vi "Array lezione operazioni.vi"() -> ()   [LabVIEW 2012]
panel:
  in  "Array":dbl[](array[numeric])
  in  "vet a":dbl[](array[numeric])=[1.0, 2.0, 3.0] format="%.2f"
  in  "vet b":dbl[](array[numeric]) format="%.2f"
  out "vet som":dbl[](array[numeric]) format="%.2f"
  in  "index select 2":i32=1
  out "index of elem.":i32=4
  in  "element":sgl format="%.2f"
  in  "start index":i32
  out "min index":i32=4
  out "min":sgl format="%.2f"
  out "max index":i32=4
  out "max":sgl format="%.2f"
  out "array cast":sgl[](array[numeric]) format="%.2f"
  in  "new element2":sgl=-2.0 format="%.2f"
  in  "new element1":sgl=3.0 format="%.2f"
  in  "lenght":i32=2
  out "array subset":sgl[](array[numeric]) format="%.2f"
  out "array out":sgl[](array[numeric]) format="%.2f"
  in  "element repl":sgl format="%.2f"
  in  "index select":i32=2
  out "element":sgl format="%.2f"
  in  "index":i32=3
  out "dim":i32=4
  in  "array in":sgl[](array[numeric])=[2.0, 4.0, 6.0, 8.0] format="%.2f"
  # "Funzioni che operano sugli array"
  # "Array Size"
  # "Index Array"
  # "Replace Array Element"
  # "Array Subset"
  # "Build Array"
  # "Array Max & Min"
  # "Search 1D Array"
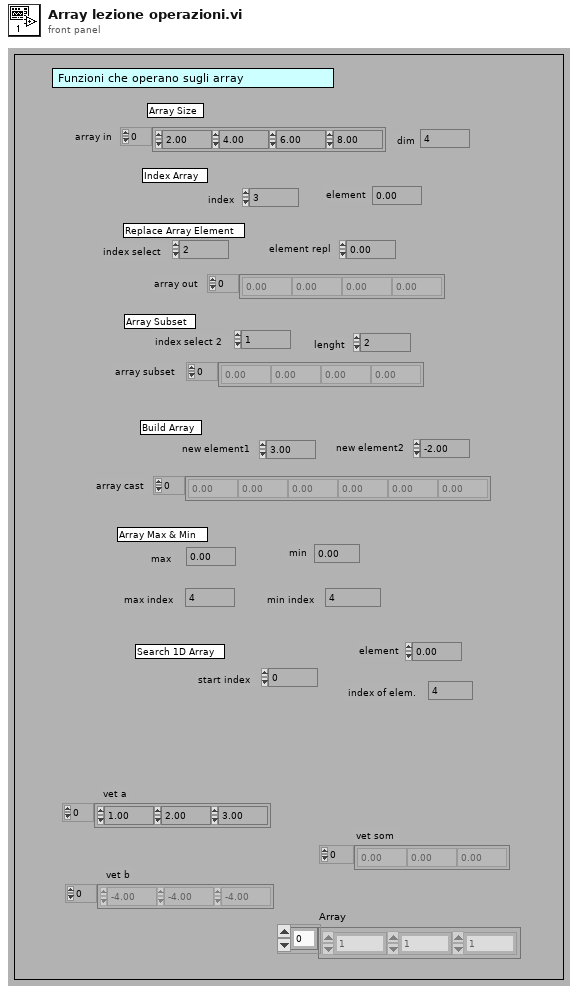
[diagram p1: front panel]
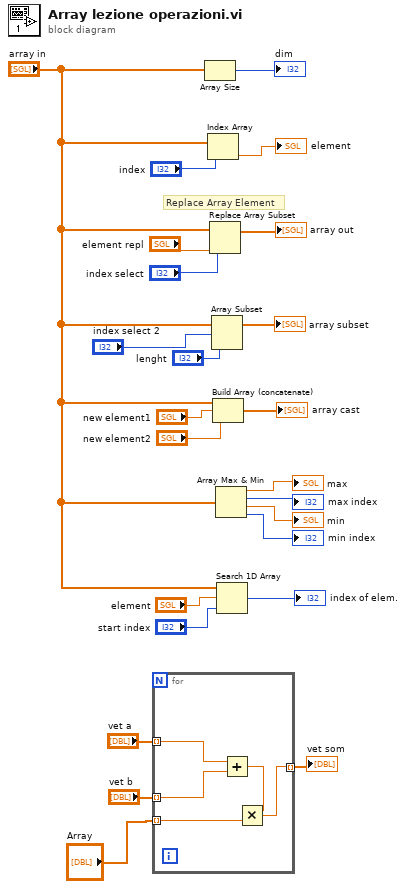
[diagram p0: block diagram]
diagram:
  # "Replace Array Element"
  n1 = for {
    tunnel: "vet a" -> [w29] mode=indexing
    tunnel: "vet b" -> [w28] mode=indexing
    tunnel: [w25] -> w4 mode=indexing
    tunnel: "Array" -> [w27] mode=indexing
    n2 = Add(x=w29, y=w28) -> (x+y=w26:dbl)
    n3 = Multiply(x=w26, y=w27) -> (x*y=w25:dbl)
  }
  "vet som" <- w4
  n4 = Array Size(array="array in") -> (size(s)=→"dim":i32)
  n5 = Index Array "Index Array"(array="array in", index="index") -> (element=→"element":sgl)
  n6 = Replace Array Subset(array="array in", new element="element repl", index="index select") -> (→"array out":sgl[])
  n7 = Array Subset "Array Subset"(array="array in", index="index select 2", length="lenght") -> (→"array subset":sgl[])
  n8 = Build Array (concatenate) "Build Array"("array in", "new element1", "new element2") -> (→"array cast":sgl[])
  n9 = Array Max & Min(array="array in") -> (max value=→"max":sgl, max index (indices)=→"max index":i32, min value=→"min":sgl, min index (indices)=→"min index":i32)
  n10 = Search 1D Array(1D array="array in", element="element", start index (0)="start index") -> (index of element=→"index of elem.":i32)
